vi "VDI Init Dig RF.vi"(7 "Speed":u16, 9 "Channel":u8, 10 "DevIndex":i32, 11 "DevType":i32) -> (3 "function return":i32)   [LabVIEW 2010, in "ControlDigRF.lvlib"]
doc: "int WINAPI VDI_InitDigRF(int DevType,int DevIndex,unsigned char Channel,unsigned short Speed);"
uses:
  ControlDigRF.lvlib
  ControlDigRF/Ginkgo_Driver.dll
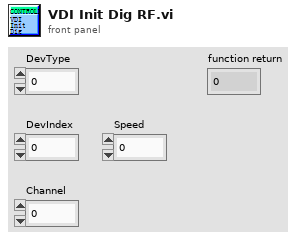
[diagram p1: front panel]
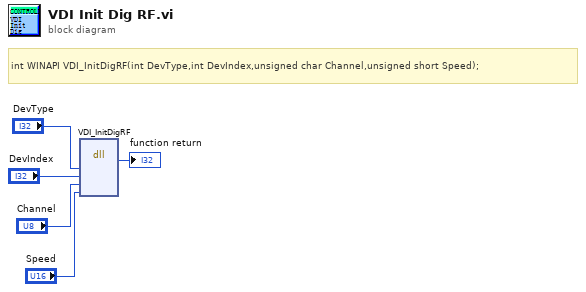
[diagram p0: block diagram]
diagram:
  # "int WINAPI VDI_InitDigRF(int DevType,int DevIndex,unsigned char Channel,unsigned short Speed);"
  n1 = dll-call lib="E:/Project/vt_ginkgo/truck/Ginkgo Driver/vs2010/Ginkgo_USB-I2C&SPI&CAN_API_v2.0.3.3/lib/labview_32bit/ControlDigRF/Ginkgo_Driver.*" fn="VDI_InitDigRF"("DevType"="DevType", "DevIndex"="DevIndex", "Channel"="Channel", "Speed"="Speed") -> (→"function return":i32)  [unwired: 7 in, 2 out]
